vi "AFM_Driver_Manager.SendBackgroundImage.vi"(8 "error in (no error)":errorcluster, 10 "Path":path, 11 "AFM_Driver_Manager in":refnum<class "AFM_Driver_Manager.lvclass">) -> (0 "error out":errorcluster, 3 "AFM_Driver_Manager out":refnum<class "AFM_Driver_Manager.lvclass">)   [LabVIEW 2019, in "AFM_Driver_Manager.lvclass"]
uses:
  AFM_Driver_Manager.lvclass
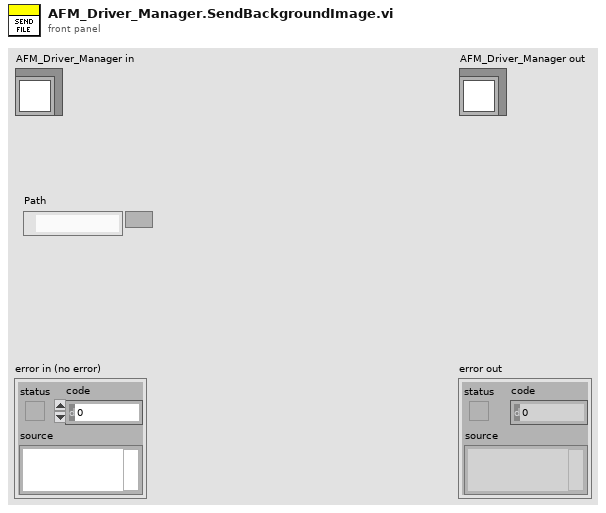
[diagram p1: front panel]
types:
  T1 = typedef "AFM_Driver_Manager.lvclass/AFM_Driver_Manager.PublicMethods.ctl" = cluster{"Stop Event":refnum<user-event>, "Lithography Data":refnum<user-event>, "Run Lithography":refnum<user-event>, "Background Image":refnum<user-event>, "Abort Notifier":refnum<user-event>}
  T2 = cluster{"VI Refnum":refnum<vi>, "Path":path, "Name":string, "Events":T1}
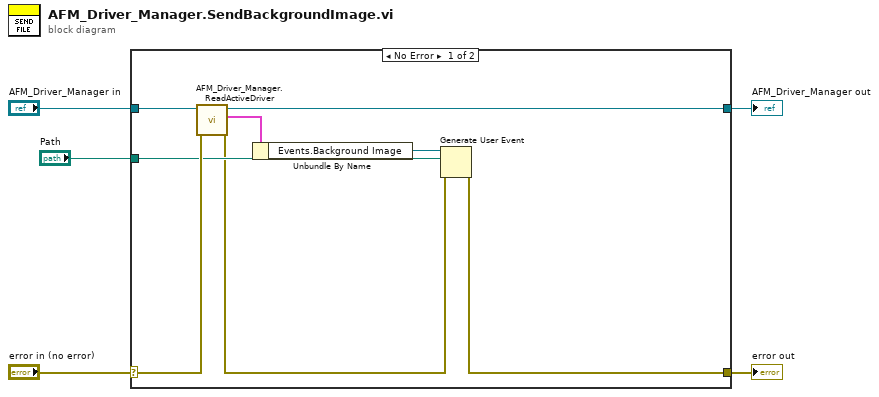
[diagram p0: block diagram]
diagram:
  n1 = case shown="No Error" "error in (no error)" {
    selector: "error in (no error)" -> [w11 w15]
    tunnel: [w6 w15] -> w4
    tunnel: [w13 w14] -> w2
    tunnel: "AFM_Driver_Manager in" -> [w12 w14]
    tunnel: "Path" -> [w8 _]
    frame No Error {
      n2 = call "AFM_Driver_Manager.ReadActiveDriver.vi"("error in (no error)"=w11, "AFM_Driver_Manager in"=w12) -> ("error out"=w7:errorcluster, "Active Driver"=w10:T2, "AFM_Driver_Manager out"=w13:refnum<class "AFM_Driver_Manager.lvclass">)  [unwired: 7 in]
      n3 = Unbundle By Name(w10) -> ("Events.Background Image"=w9:refnum<user-event>)
      n4 = Generate User Event(user event=w9, event data cluster=w8, error in=w7) -> (error out=w6:errorcluster)  [unwired: 1 in, 1 out]
    }
    frame Error {
    }
  }
  "error out" <- w4
  "AFM_Driver_Manager out" <- w2
